vi "CreateExerciseConfiguration.vi"(11 "Exercise Number":u32) -> (0 "Wfm Type":T1=enum."Chirp", 3 "Exercise Configuration":T2)   [LabVIEW 2014]
uses:
  Ctls/ExerciseWfmType.ctl
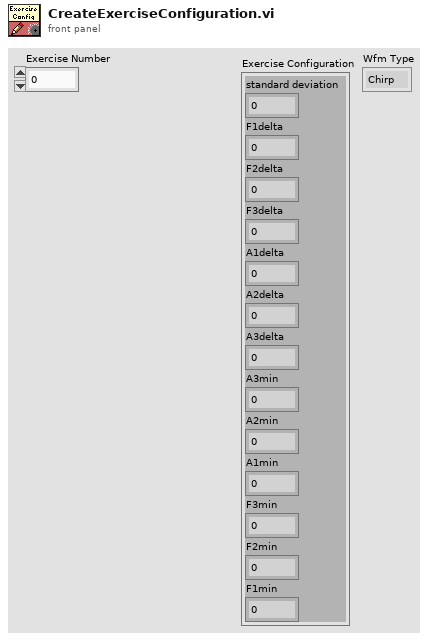
[diagram p1: front panel]
types:
  T1 = typedef "ExerciseWfmType.ctl" = enum16{"Multitone", "Chirp"}
  T2 = cluster{"standard deviation":dbl, "F1delta":dbl, "F2delta":dbl, "F3delta":dbl, "A1delta":dbl, "A2delta":dbl, "A3delta":dbl, "A3min":dbl, "A2min":dbl, "A1min":dbl, "F3min":dbl, "F2min":dbl, "F1min":dbl}
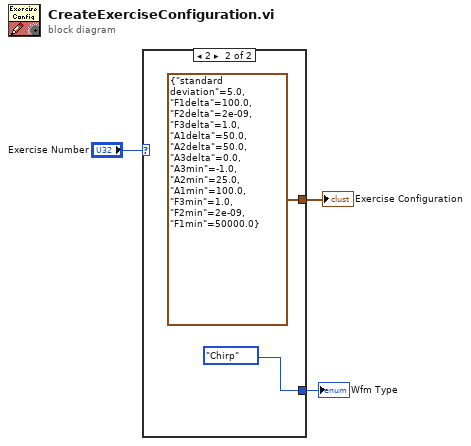
[diagram p0: block diagram]
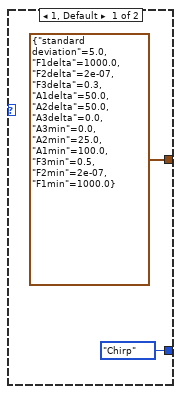
[diagram p2: hidden frame]
diagram:
  n1 = case shown="2" "Exercise Number" {
    tunnel: [T2 {"standard deviation"=5.0, "F1delta"=1000.0, "F2delta"=2e-07, "F3delta"=0.3, "A1delta"=50.0, "A2delta"=50.0, "A3delta"=0.0, "A3min"=0.0, "A2min"=25.0, "A1min"=100.0, "F3min"=0.5, "F2min"=2e-07, "F1min"=1000.0} ("F & A") T2 {"standard deviation"=5.0, "F1delta"=100.0, "F2delta"=2e-09, "F3delta"=1.0, "A1delta"=50.0, "A2delta"=50.0, "A3delta"=0.0, "A3min"=-1.0, "A2min"=25.0, "A1min"=100.0, "F3min"=1.0, "F2min"=2e-09, "F1min"=50000.0} ("F & A")] -> w3
    tunnel: [ExerciseWfmType."Chirp" ("Enum") ExerciseWfmType."Chirp" ("Enum")] -> w2
    frame 1, Default {
    }
    frame 2 {
    }
  }
  "Exercise Configuration" <- w3
  "Wfm Type" <- w2
